vi "操作日志.vi"(8 "error in (no error)":errorcluster, 10 "table":string="操作日志", 11 "日志信息":string) -> (0 "error out":errorcluster)   [LabVIEW 2016, in "斯坦道多参数.lvlib"]
uses:
  <vilib>/Utility/sysdir.llb/System Directory Type.ctl
  <vilib>/addons/database/Connection.llb/DB Tools Open Connec (String).vi
  <vilib>/addons/database/NI_Database_API.lvlib
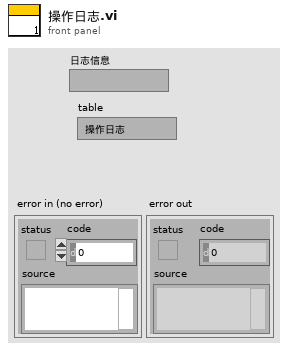
[diagram p1: front panel]
types:
  T1 = cluster{"时间标识":timestamp, "设备":string, "日志信息":string, "流程参数":string}
  T2 = typedef "System Directory Type.ctl" = i32
  T3 = typedef "NI_Database_API.lvlib/Conn ObjectReference.ctl" = refnum<k1>
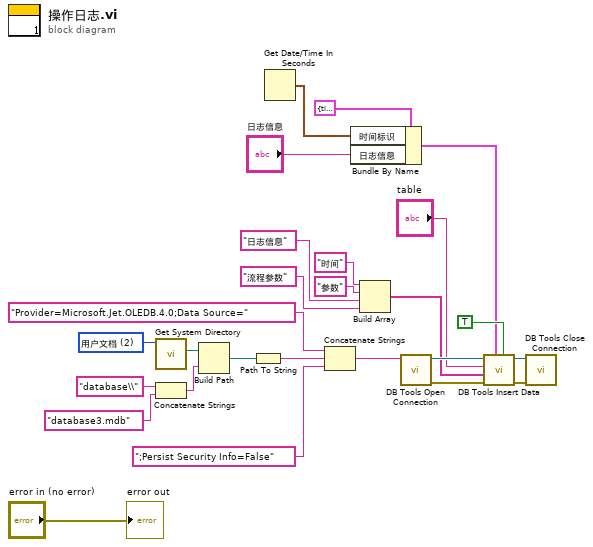
[diagram p0: block diagram]
diagram:
  w19 = T2 2 items=["用户目录"=0, "用户桌面"=1, "用户文档"=2, "用户应用程序数据"=3, "用户设置"=4, "用户临时目录"=5, "公共文档"=6, "公共应用程序数据"=7, "公共设置"=8, "公共缓存"=13, "系统核心库"=9, "系统安装库"=10, "应用程序文件"=11, "启动盘根目录"=12] ("system directory type")
  n1 = call <vilib>:"Get System Directory.vi"("system directory type"=w19) -> ("system directory"=w17:path)  [unwired: 10 in]
  n2 = Concatenate Strings("database\\" ("condition"), "database3.mdb" ("database")) -> (w11:string)
  n3 = Build Path(base path=w17, name or relative path=w11) -> (appended path=w16:path)
  n4 = Path To String(path=w16) -> (string=w15:string)
  n5 = Get Date/Time In Seconds() -> (seconds since 1Jan1904=w3:timestamp)
  n6 = Concatenate Strings("Provider=Microsoft.Jet.OLEDB.4.0;Data Source=" ("condition"), w15, ";Persist Security Info=False" ("condition")) -> (w13:string)
  n7 = Bundle By Name(cluster=T1 {"时间标识"=timestamp(0 s since 1904-01-01), "设备"="多参数", "日志信息"="", "流程参数"=""} ("data in"), "时间标识"=w3, "日志信息"="日志信息") -> (w2:T1)
  n8 = Build Array("时间", "参数" ("元素"), "日志信息", "流程参数") -> (w6:string[])
  n9 = call-poly <vilib>:"DB Tools Open Connection.vi"("connection information"=w13) -> ("error out"=w9:errorcluster, "connection reference"=w10:T3)  [unwired: 7 in]
  n10 = call <vilib>:"DB Tools Insert Data.vi"("create table? (F)"=TRUE, "data"=w2, "error in (no error)"=w9, "columns"=w6, "table"="table", "connection reference"=w10) -> ("error out"=w21:errorcluster, "connection reference out"=w22:T3)  [unwired: 4 in]
  n11 = call <vilib>:"DB Tools Close Connection.vi"("error in (no error)"=w21, "connection reference"=w22) -> ()  [unwired: 5 in, 1 out]
  "error out" <- "error in (no error)"
